vi "average_num.vi"() -> ()   [LabVIEW 2020]
panel:
  in  "stop":bool
  out "Exceeding\ntheshold":bool
  out "average_gauge":dbl(knob) scale=0.0..10.0
  out "average_thermo":dbl(slide) scale=0.0..100.0
  out "average_meter":dbl(knob) scale=0.0..10.0
  out "average_num":dbl
  in  "num5":dbl(knob) scale=0.0..10.0
  in  "num3":dbl(slide) scale=0.0..10.0
  in  "num2":dbl(slide) scale=0.0..10.0
  in  "num1":dbl
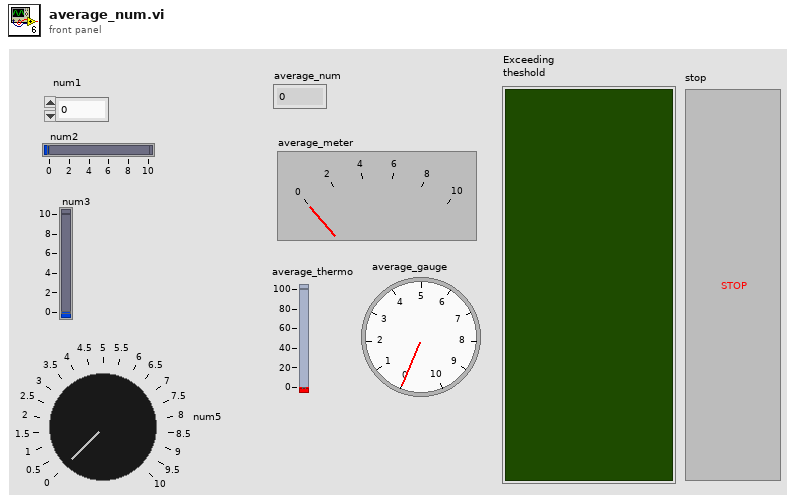
[diagram p1: front panel]
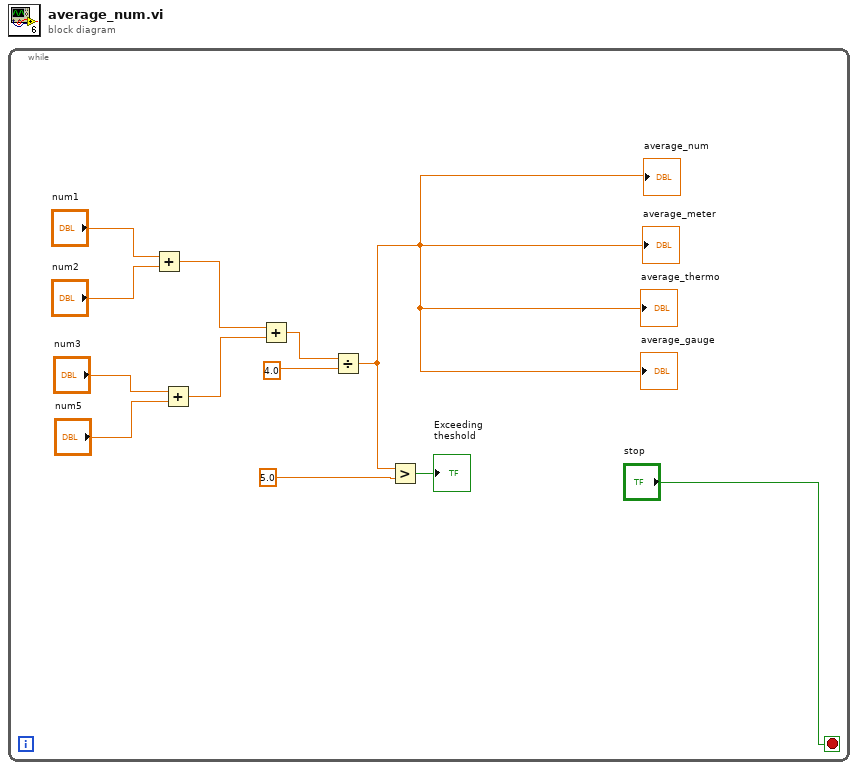
[diagram p0: block diagram]
diagram:
  n1 = while {
    stop <- "stop" stop-if-true
    n2 = Add(x="num1", y="num2") -> (x+y=w8:dbl)
    n3 = Add(x="num3", y="num5") -> (x+y=w7:dbl)
    n4 = Add(x=w8, y=w7) -> (x+y=w6:dbl)
    n5 = Divide(x=w6, y=4.0) -> (x/y=w2:dbl)
    "average_num" <- w2
    "average_meter" <- w2
    "average_thermo" <- w2
    "average_gauge" <- w2
    n6 = Greater?(x=w2, y=5.0) -> (0:→"Exceeding\ntheshold":bool)
  }
